vi "Read Name.vi"(11 "Log Sink in":refnum<class "Log Sink.lvclass">) -> (2 "Name":string, 3 "Log Sink out":refnum<class "Log Sink.lvclass">)   [LabVIEW 2018, in "MVA Framework.lvlib" / "Composed Log.lvlib" / "Log Sink.lvclass"]
uses:
  Log Sink.lvclass
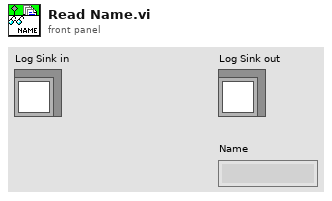
[diagram p1: front panel]
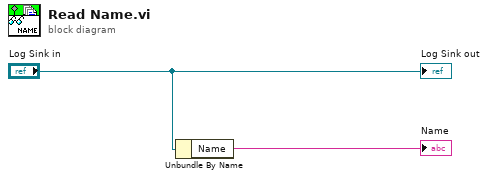
[diagram p0: block diagram]
diagram:
  n1 = Unbundle By Name("Log Sink in") -> ("Name"=→"Name":string)
  "Log Sink out" <- "Log Sink in"
